vi "Tester.vi"   [LabVIEW 2019]
uses:
  GOOP Probe/GOOP Probe.lvlib
  Child_class/Child.lvclass
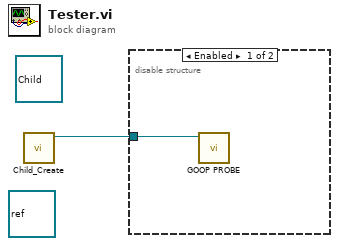
[diagram p0: block diagram]
diagram:
  (unwired) refnum<class> refnum ("LabVIEW Object")
  (unwired) refnum<class "Child.lvclass"> refnum ("reference in")
  n1 = call "Child_Create.vi"() -> ("reference out"=w1:refnum<class "Child.lvclass">)  [unwired: 10 in, 1 out]
  n2 = disable-structure shown="Enabled" {
    disable-tunnel: w1 -> [w2 _]
    frame Enabled {
      n3 = call "GOOP PROBE.vi"("Probed Object"=w2) -> ()  [unwired: 9 in, 2 out]
    }
    frame Disabled {
    }
  }
